vi "Launcher.vi"() -> ()   [LabVIEW 2024]
uses:
  Test_class/Test.lvclass
  <vilib>/Utility/miscctls.llb/LVRectTypeDef.ctl
  PositionPositionTest_class/PositionPositionTest.lvclass
  C:/Users/burakkorkmaz/Desktop/Leveling/labview-desing-patterns/Template Method Pattern/Test_class/Test.lvclass
  PositionSpeedTest_class/PositionSpeedTest.lvclass
  SpeedTorqueTest_class/SpeedTorqueTest.lvclass
  C:/Users/burakkorkmaz/Desktop/Leveling/labview-desing-patterns/Template Method Pattern/PositionPositionTest_class/PositionPositionTest.lvclass
  C:/Users/burakkorkmaz/Desktop/Leveling/labview-desing-patterns/Template Method Pattern/PositionSpeedTest_class/PositionSpeedTest.lvclass
  C:/Users/burakkorkmaz/Desktop/Leveling/labview-desing-patterns/Template Method Pattern/SpeedTorqueTest_class/SpeedTorqueTest.lvclass
panel:
  in  "Repeat":u16=1
  in  "Dyno":bool
  in  "Engine":bool
  in  "Start Button":bool
  in  "Test Selector":T1(ring)
  out "History":string
  # "360x400"
  # "Test Type"
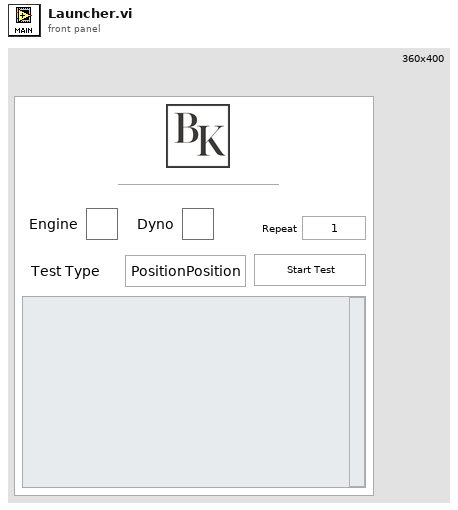
[diagram p1: front panel]
types:
  T1 = enum16{"PositionPosition", "PositionSpeed", "SpeedTorque"}
  T2 = typedef "LVRectTypeDef.ctl" = cluster{"Left":i16, "Top":i16, "Right":i16, "Bottom":i16}
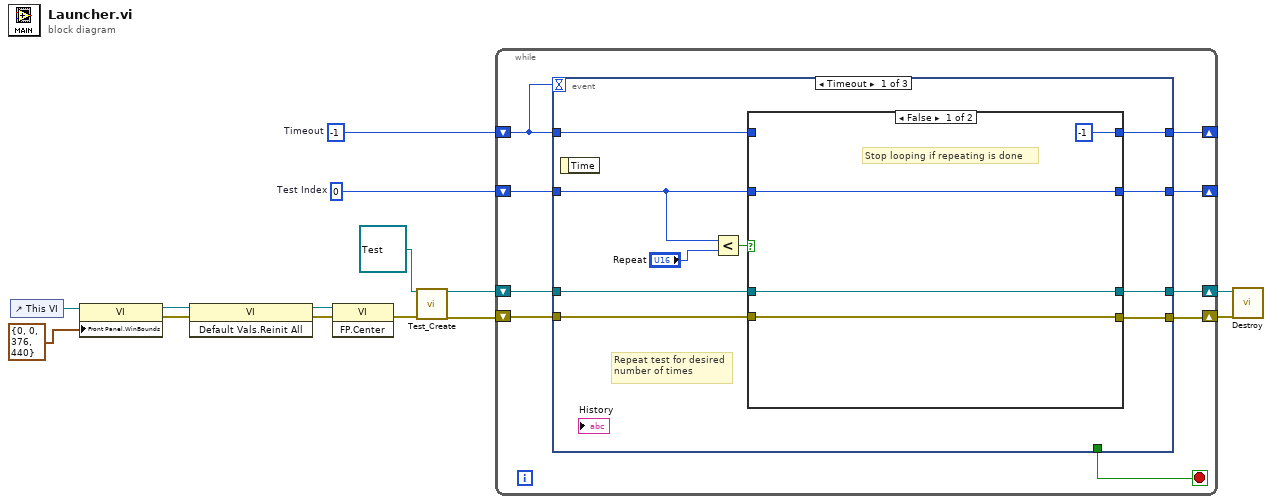
[diagram p0: block diagram]
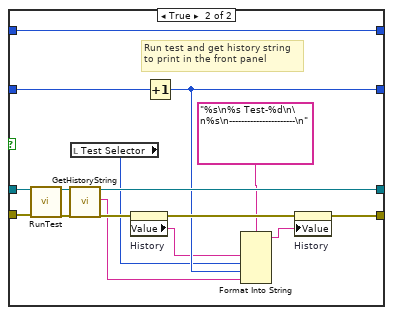
[diagram p2: hidden frame]
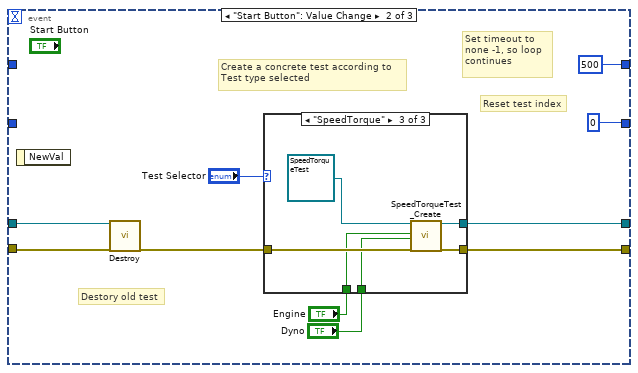
[diagram p3: hidden frame]
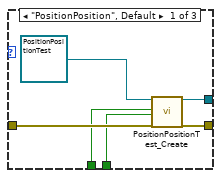
[diagram p4: hidden frame]
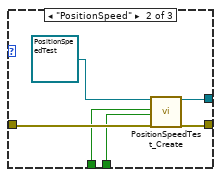
[diagram p5: hidden frame]
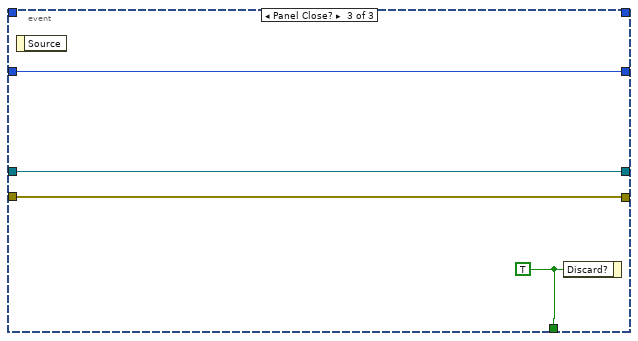
[diagram p6: hidden frame]
diagram:
  w8 = u16 0  # Test Index
  w13 = -1  # Timeout
  n1 = control-ref of="This VI"() -> (w7:refnum<vi>)
  n2 = property class="VI"(reference=w7, "Front Panel.WinBounds"=T2 {"Left"=0, "Top"=0, "Right"=376, "Bottom"=440} ("Front Panel Window:Window Bounds")) -> (reference out=w6:refnum<vi>, error out=w4:errorcluster)  [unwired: 1 in]
  n3 = invoke class="VI" method="Default Vals.Reinit All"(reference=w6, error in=w4) -> (reference out=w5:refnum<vi>, error out=w3:errorcluster)  [unwired: 1 in, 1 out]
  n4 = invoke class="VI" method="FP.Center"(reference=w5, error in=w3) -> (error out=w1:errorcluster)  [unwired: 1 in, 2 out]
  n5 = call "Test_Create.vi"("reference in"=refnum<class "Test.lvclass"> refnum ("Test"), "error in (no error)"=w1) -> ("reference out"=w12:refnum<class "Test.lvclass">, "error out"=w11:errorcluster)  [unwired: 16 in]
  n6 = while {
    shift-right: [w22] -> w9
    shift-left: w12 -> [w21]
    shift-right: [w19] -> w10
    shift-left: w11 -> [w20]
    shift-right: [w18] -> _
    shift-left: w13 -> [w15]
    shift-right: [w16] -> _
    shift-left: w8 -> [w17]
    stop <- w23 stop-if-true
    n7 = event shown="[0] Timeout" {
      selector: _ -> [_ _ _]
      dyn-events: _ -> [_ _ _]
      timeout: w15 -> [_ _ _]
      tunnel: [_ _ w85] -> w23
      tunnel: [w30 w62 w84] -> w22
      tunnel: w21 -> [w33 w61 w84]
      tunnel: w20 -> [w32 w60 w83]
      tunnel: [w31 w57 w83] -> w19
      tunnel: [w25 500 _] -> w18
      tunnel: w17 -> [w27 _ w82]
      tunnel: [w26 u16 0 w82] -> w16
      tunnel: w15 -> [w24 _ _]
      event Timeout {
        # "Repeat test for desired\nnumber of times"
        n8 = event-data() -> ()  [unwired: 1 in, 1 out]
        n9 = Less?(x=w27, y="Repeat") -> (x < y?=w29:bool)
        n10 = case shown="False" w29 {
          tunnel: w33 -> [w37 w53]
          tunnel: w32 -> [w36 w52]
          tunnel: [w36 w45] -> w31
          tunnel: [w37 w49] -> w30
          tunnel: w27 -> [w35 w48]
          tunnel: [w35 w40] -> w26
          tunnel: [-1 w44] -> w25
          tunnel: w24 -> [_ w44]
          frame False {
            # "Stop looping if repeating is done"
          }
          frame True {
            # "Run test and get history string\nto print in the front panel"
            n11 = call-dynamic "RunTest.vi"("reference in"=w53, "error in (no error)"=w52) -> ("reference out"=w50:refnum<class "Test.lvclass">, "error out"=w51:errorcluster)  [unwired: 16 in]
            n12 = call-dynamic "GetHistoryString.vi"("reference in"=w50, "error in (no error)"=w51) -> ("reference out"=w49:refnum<class "Test.lvclass">, "History String"=w41:string, "error out"=w47:errorcluster)  [unwired: 15 in]
            n13 = local read "Test Selector"() -> (w38:T1)
            n14 = property on="History" class="Str"(error in=w47) -> (error out=w46:errorcluster, "Value"=w39:string)  [unwired: 1 in, 1 out]
            n15 = Increment(x=w48) -> (x+1=w40:u16)
            n16 = Format Into String(format string="%s\n%s Test-%d\n\n%s\n----------------------\n", w39, w38, w40, w41) -> (resulting string=w42:string)  [unwired: 2 in, 1 out]
            n17 = property on="History" class="Str"(error in=w46, "Value"=w42) -> (error out=w45:errorcluster)  [unwired: 1 in, 1 out]
          }
        }
      }
      event "Start Button": Value Change {
        # "Destory old test"
        # "Reset test index"
        # "Set timeout to\nnone -1, so loop\ncontinues"
        # "Create a concrete test according to\nTest type selected"
        n18 = event-data() -> ()  [unwired: 1 in, 1 out]
        n19 = call-dynamic "Destroy.vi"("reference in"=w61, "error in (no error)"=w60) -> ("error out"=w58:errorcluster)  [unwired: 16 in, 1 out]
        n20 = case shown="\"SpeedTorque\"" "Test Selector" {
          tunnel: [w68 w75 w81] -> w62
          tunnel: w58 -> [w67 w73 w79]
          tunnel: [w66 w74 w80] -> w57
          tunnel: "Engine" -> [w65 w71 w77]
          tunnel: "Dyno" -> [w64 w70 w76]
          frame "PositionPosition", Default {
            n21 = call "PositionPositionTest_Create.vi"("reference in"=refnum<class "PositionPositionTest.lvclass"> refnum ("PositionPositionTest"), "Engine"=w65, "Dyno"=w64, "error in (no error)"=w67) -> ("reference out"=w68:refnum<class "PositionPositionTest.lvclass">, "error out"=w66:errorcluster)  [unwired: 14 in]
          }
          frame "PositionSpeed" {
            n22 = call "PositionSpeedTest_Create.vi"("reference in"=refnum<class "PositionSpeedTest.lvclass"> refnum ("PositionSpeedTest"), "Engine"=w71, "Dyno"=w70, "error in (no error)"=w73) -> ("reference out"=w75:refnum<class "PositionSpeedTest.lvclass">, "error out"=w74:errorcluster)  [unwired: 14 in]
          }
          frame "SpeedTorque" {
            n23 = call "SpeedTorqueTest_Create.vi"("reference in"=refnum<class "SpeedTorqueTest.lvclass"> refnum ("SpeedTorqueTest"), "Engine"=w77, "Dyno"=w76, "error in (no error)"=w79) -> ("reference out"=w81:refnum<class "SpeedTorqueTest.lvclass">, "error out"=w80:errorcluster)  [unwired: 14 in]
          }
        }
      }
      event Panel Close? {
        w85 = TRUE ("Discard?")
        n24 = event-data() -> ()  [unwired: 1 in, 1 out]
        n25 = event-data("Discard?"=w85) -> ()  [unwired: 1 in, 1 out]
      }
    }
  }
  n26 = call-dynamic "Destroy.vi"("reference in"=w9, "error in (no error)"=w10) -> ()  [unwired: 16 in, 2 out]
